vi "TB-Initialize Analysis.vi"(0 "Analysis":T2, 5 "imic":i32, 7 "isig":i32, 9 "Fs (Hz)":dbl, 11 "Buffer length (s)":dbl) -> (8 "state":T1)   [LabVIEW 2020]
uses:
  Typedefs/TB-Analysis Parameters.ctl
  Typedefs/TB-Analysis State.ctl
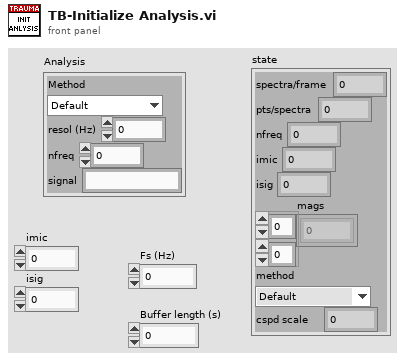
[diagram p1: front panel]
types:
  T1 = typedef "TB-Analysis State.ctl" = cluster{"spectra/frame":i32, "pts/spectra":i32, "nfreq":i32, "imic":i32, "isig":i32, "mags":dbl[][], "method":enum16{"Default", "Periodogram", "Cross-spectrum"}, "cspd scale":dbl}
  T2 = typedef "TB-Analysis Parameters.ctl" = cluster{"Method":enum16{"Default", "Periodogram", "Cross-spectrum"}, "resol (Hz)":dbl, "nfreq":i32, "signal":string}
  T3 = enum16{"Default", "Periodogram", "Cross-spectrum"}
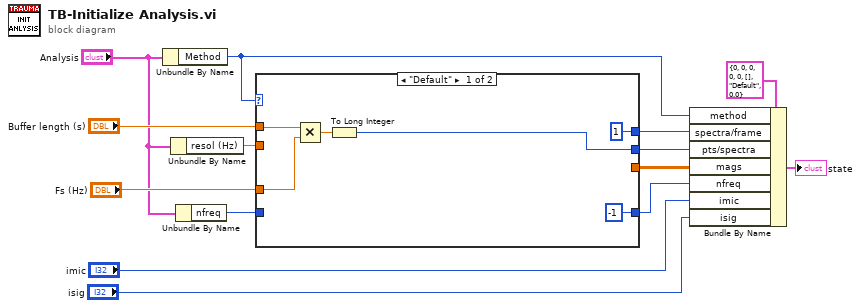
[diagram p0: block diagram]
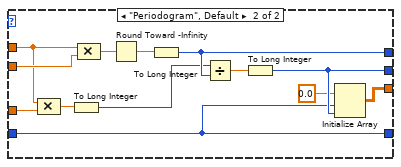
[diagram p2: hidden frame]
diagram:
  n1 = Unbundle By Name("Analysis") -> ("Method"=w1:T3)
  n2 = Unbundle By Name("Analysis") -> ("resol (Hz)"=w14:dbl)
  n3 = Unbundle By Name("Analysis") -> ("nfreq"=w10:i32)
  n4 = case shown="\"Default\"" w1 {
    tunnel: w14 -> [_ w31]
    tunnel: [1 w30] -> w8
    tunnel: "Buffer length (s)" -> [w18 w29]
    tunnel: "Fs (Hz)" -> [w17 w28]
    tunnel: [w15 w24] -> w7
    tunnel: w10 -> [_ w21]
    tunnel: [_ w22] -> w6
    tunnel: [-1 ("nfreq") w21] -> w5
    frame "Default" {
      n5 = Multiply(x=w18, y=w17) -> (x*y=w16:dbl)
      n6 = To Long Integer(number=w16) -> (32bit integer=w15:i32)
    }
    frame "Periodogram", Default {
      n7 = Compound Arithmetic op=MULTIPLY(w29, w28) -> (w27:dbl)
      n8 = To Long Integer(number=w27) -> (32bit integer=w25:i32)
      n9 = Compound Arithmetic op=MULTIPLY(w29, w31) -> (w33:dbl)
      n10 = Round Toward -Infinity(1:w33) -> (0:w32:dbl)
      n11 = To Long Integer(number=w32) -> (32bit integer=w30:i32)
      n12 = Divide(x=w25, y=w30) -> (x/y=w26:dbl)
      n13 = To Long Integer(number=w26) -> (32bit integer=w24:i32)
      n14 = Initialize Array(0.0, w21, w24) -> (w22:dbl[][])
    }
  }
  n15 = Bundle By Name(cluster=T1 {"spectra/frame"=0, "pts/spectra"=0, "nfreq"=0, "imic"=0, "isig"=0, "mags"=[], "method"=enum."Default", "cspd scale"=0.0} ("state"), "method"=w1, "spectra/frame"=w8, "pts/spectra"=w7, "mags"=w6, "nfreq"=w5, "imic"="imic", "isig"="isig") -> (→"state":T1)
